vi "Manejo_basico_LabView.vi"() -> ()   [LabVIEW 2014]
uses:
  <vilib>/LabVIEW Interface for Arduino/Type Defs/Board Type.ctl
  <vilib>/LabVIEW Interface for Arduino/Type Defs/Pin Mode.ctl
  <vilib>/LabVIEW Interface for Arduino/LabVIEW Interface for Arduino.lvlib
panel:
  out "Boolean":bool
  in  "stop":bool
  out "Waveform Chart":dbl(graph)
  out "Voltage":dbl(knob) scale=0.0..5.0
  in  "Board Type (Mega)":T1
  in  "VISA resource":refnum<visa-resource-name>
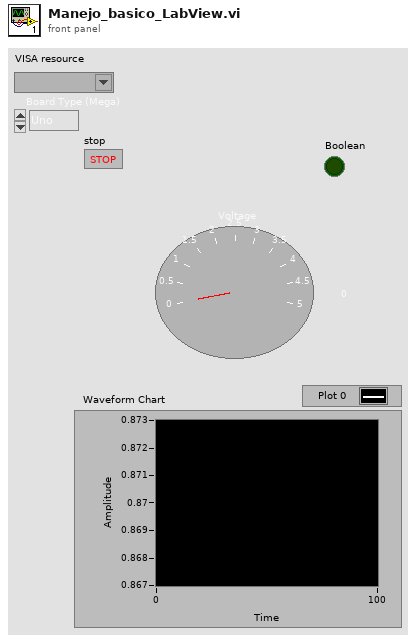
[diagram p1: front panel]
types:
  T1 = typedef "LabVIEW Interface for Arduino.lvlib/Board Type.ctl" = enum16{"Uno", "Dimuelanove w/Atmega 328", "Mega 2560"}
  T2 = typedef "LabVIEW Interface for Arduino.lvlib/Arduino Resource.ctl" = cluster{"VISA resource":refnum<visa-resource-name>, "Board Type":T1, "Connection Type":enum8{"USB / Serial"}, "Bytes Per Packet (15)":u8}
  T3 = typedef "LabVIEW Interface for Arduino.lvlib/Pin Mode.ctl" = enum8{"Input", "Output"}
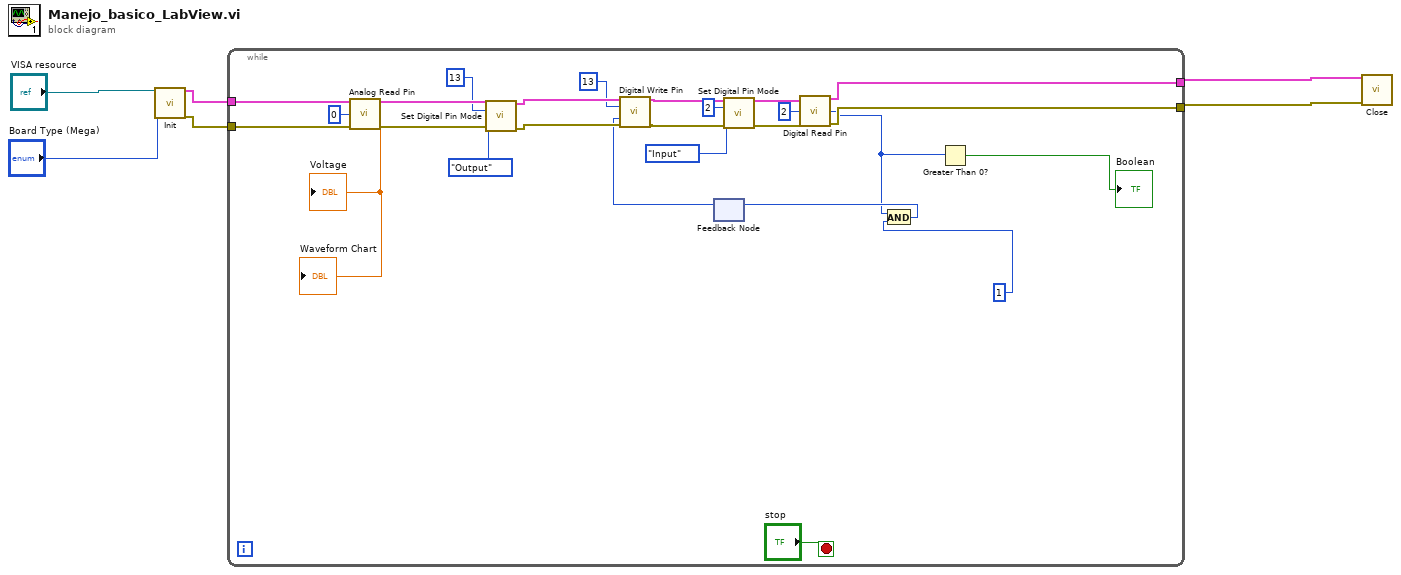
[diagram p0: block diagram]
diagram:
  n1 = call <vilib>:"Init.vi"("VISA resource"="VISA resource", "Board Type (Uno)"="Board Type (Mega)") -> ("Arduino Resource"=w4:T2, "error out"=w2:errorcluster)  [unwired: 16 in]
  n2 = while {
    tunnel: w4 -> [w32]
    tunnel: [w15] -> w3
    tunnel: w2 -> [w29]
    tunnel: [w13] -> w1
    stop <- "stop" stop-if-true
    n3 = call <vilib>:"Analog Read Pin.vi"("Arduino Resource"=w32, "Analog Input Pin (0)"=u8 0, "error in"=w29) -> ("Arduino Resource"=w31:T2, "Voltage"=→"Voltage" →"Waveform Chart":dbl, "error out"=w28:errorcluster)  [unwired: 10 in]
    n4 = call <vilib>:"Set Digital Pin Mode.vi"("Arduino Resource"=w31, "Digital I/O Pin"=u8 13, "Pin Mode (Input)"=Pin_Mode."Output", "error in"=w28) -> ("Arduino Resource"=w30:T2, "error out"=w27:errorcluster)  [unwired: 10 in]
    n5 = feedback #1() -> (w9:i32)  [unwired: 1 in]
    n6 = call <vilib>:"Digital Write Pin.vi"("Arduino Resource"=w30, "Digital I/O Pin (0)"=u8 13, "Value (0)"=w9, "error in"=w27) -> ("Arduino Resource"=w20:T2, "error out"=w19:errorcluster)  [unwired: 10 in]
    n7 = call <vilib>:"Set Digital Pin Mode.vi"("Arduino Resource"=w20, "Digital I/O Pin"=u8 2, "Pin Mode (Input)"=Pin_Mode."Input", "error in"=w19) -> ("Arduino Resource"=w16:T2, "error out"=w14:errorcluster)  [unwired: 10 in]
    n8 = call <vilib>:"Digital Read Pin.vi"("Arduino Resource"=w16, "Digital I/O Pin (0)"=u8 2, "error in"=w14) -> ("Arduino Resource"=w15:T2, "Value"=w8:u8, "error out"=w13:errorcluster)  [unwired: 10 in]
    n9 = And(x=w8, y=1) -> (x .and. y?=w10:i32)
    n10 = feedback-in #1(w10) -> ()
    n11 = Greater Than 0?(x=w8) -> (x > 0?=→"Boolean":bool)
  }
  n12 = call <vilib>:"Close.vi"("Arduino Resource"=w3, "error in"=w1) -> ()  [unwired: 13 in, 1 out]
